vi "Read From Spreadsheet File.vi"(4 "delimiter (Tab)":string="\t" caption="Trennzeichen (Tab)", 6 "transpose (no:F)":bool caption="Transponieren (nein:F)", 7 "format (%.3f)":string="%.3f" caption="Format (%.3f)", 8 "max characters/row  (no limit:0)":i32 caption="Max. Zeichen pro Zeile  (keine Begrenzung:0)", 9 "start of read offset (chars.:0)":i32 caption="Position Lese-Offset (chars.: 0)", 10 "number of rows (all:-1)":i32=-1 caption="Anzahl Reihen (alle:-1)", 11 "file path (dialog if empty)":path caption="Dateipfad (Dialog, wenn leer)") -> (0 "EOF?":bool caption="Dateiende?", 1 "mark after read (chars.)":i32 caption="Dateimarke nach Lesevorgang (Zeichen)", 2 "first row":sgl[](array[numeric]) caption="Erste Zeile" format="%0.3f", 3 "all rows":sgl[][](array[numeric]) caption="Alle Zeilen" format="%0.3f", 5 "new file path (Not A Path if cancelled)":path caption="Neuer Dateipfad (Kein Pfad, wenn abgebrochen)")   [LabVIEW 2009]
doc: "Liest eine festgelegte Anzahl von Zeilen einer numerischen Textdatei beginnend am angegebenen Zeichen-Offset und konvertiert die Daten in ein 2D-Array mit Fließkommazahlen einfacher Genauigkeit."
panel:
  in  "type (empty)":sgl[][](array[numeric]) caption="Typ (leer)" format="%0.2f"
  # "Zeilen\nSpalten"
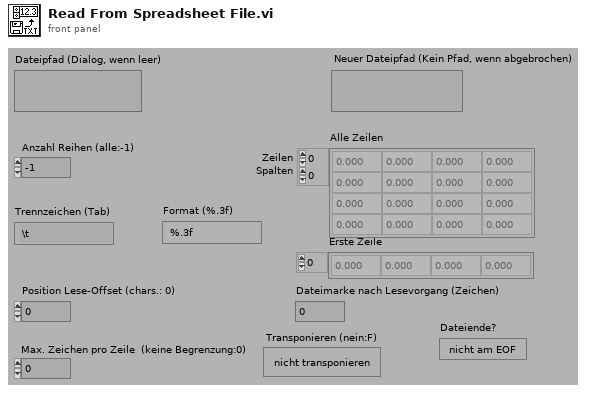
[diagram p1: front panel]
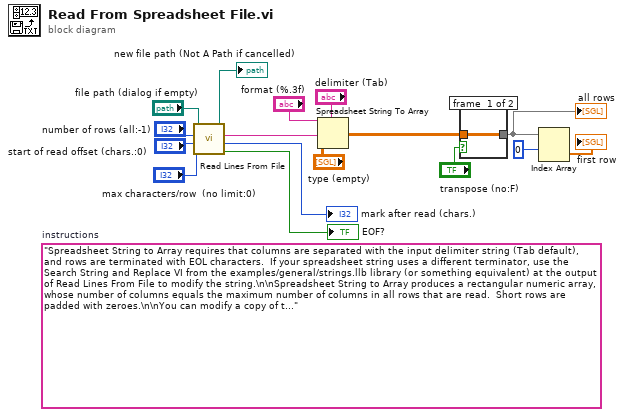
[diagram p0: block diagram]
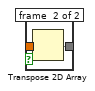
[diagram p2: hidden frame]
diagram:
  (unwired) "Spreadsheet String to Array requires that columns are separated with the input delimiter string (Tab default), and rows are terminated with EOL characters.  If your spreadsheet string uses a different terminator, use the Search String and Replace VI from the examples/general/strings.llb library (or something equivalent) at the output of Read Lines From File to modify the string.\n\nSpreadsheet String to Array produces a rectangular numeric array, whose number of columns equals the maximum number of columns in all rows that are read.  Short rows are padded with zeroes.\n\nYou can modify a copy of this VI to return the file contents into arrays of strings by changing all rows, first row, and type (empty) arrays to string arrays and by setting the format to %s."  # instructions
  n1 = call "Read Lines From File.vi"("file path (dialog if empty)"="file path (dialog if empty)", "number of lines (all:-1)"="number of rows (all:-1)", "start of read offset (chars.:0)"="start of read offset (chars.:0)", "[max characters per line]  (no limit:0)"="max characters/row  (no limit:0)") -> ("new file path (Not A Path if cancelled)"=→"new file path (Not A Path if cancelled)":path, "line string"=w12:string, "mark after read (chars.)"=→"mark after read (chars.)":i32, "EOF?"=→"EOF?":bool)  [unwired: 2 in]
  n2 = Spreadsheet String To Array(delimiter (Tab)="delimiter (Tab)", format string="format (%.3f)", spreadsheet string=w12, array type (2D Dbl)="type (empty)") -> (array=w10:sgl[][])
  n3 = case shown="True" "transpose (no:F)" {
    tunnel: [w17 w19] -> w7
    tunnel: w10 -> [w17 w18]
    frame #0 {
    }
    frame #1 {
      n4 = Transpose 2D Array(2D array=w18) -> (transposed array=w19:sgl[][])
    }
  }
  "all rows" <- w7
  n5 = Index Array(array=w7, index (row)=0) -> (element=→"first row":sgl[])  [unwired: 1 in]
